vi "get text after first open bracket.vi"(1 "Python String":string) -> (0 "Text After First Open Bracket":string)   [LabVIEW 2020, in "jki_python_data_tools.lvlib"]
uses:
  jki_python_data_tools.lvlib
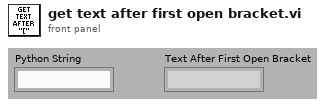
[diagram p1: front panel]
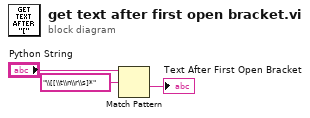
[diagram p0: block diagram]
diagram:
  n1 = Match Pattern(string="Python String", regular expression="\\[[\\t\\n\\r\\s]*") -> (after substring=→"Text After First Open Bracket":string)  [unwired: 1 in, 3 out]
